vi "Initialize UDP Configuration.vi"(8 "error in (no error)":errorcluster, 11 "UDP Configuration in":refnum<class "UDP Configuration.lvclass">) -> (0 "error out":errorcluster, 3 "UDP Configuration out":refnum<class "UDP Configuration.lvclass">)   [LabVIEW 2017, in "UDP Transceiver.lvlib" / "UDP Configuration.lvclass"]
uses:
  UDP Configuration.lvclass
  C:/DSF/Core/Data Sharing Framework Core.lvlibp/Engine/Internal/Configuration Classes/Configuration/Configuration.lvclass
  UDP Configuration.lvclass/UDP Configuration.ctl
  DSF/Core/Data Sharing Framework Core.lvlibp/Engine/Internal/Configuration Classes/Configuration/Configuration.lvclass
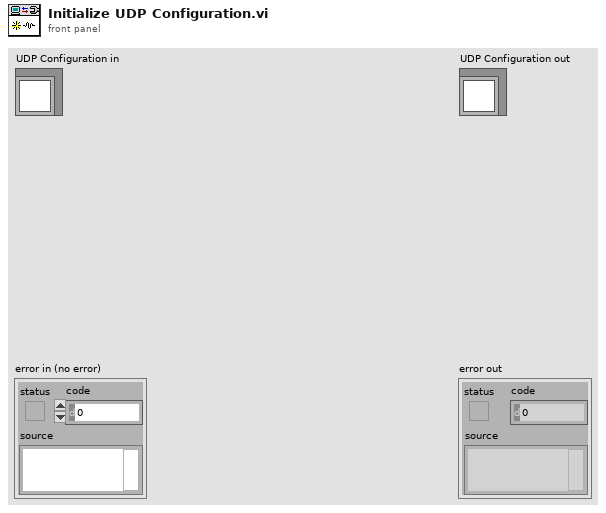
[diagram p1: front panel]
types:
  T1 = typedef "Data Sharing Framework Core.lvlibp/Data Sharing Framework Configuration.lvlib/DSF Settings Info.ctl" = cluster{"key":string, "value":string}[]
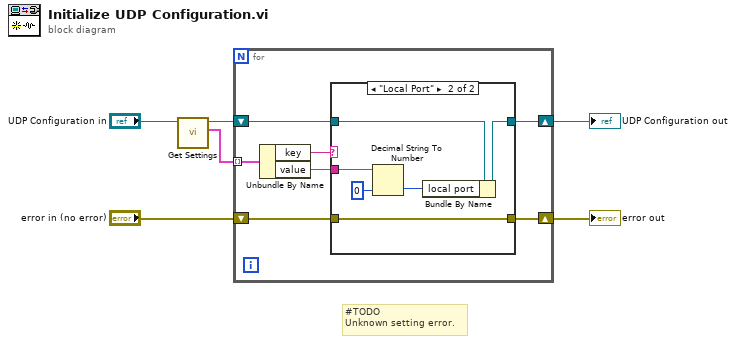
[diagram p0: block diagram]
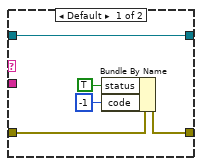
[diagram p2: hidden frame]
diagram:
  # "#TODO\nUnknown setting error."
  n1 = call "Get Settings.vi"("Configuration in"="UDP Configuration in") -> ("settings"=w5:T1, "Configuration out"=w4:refnum<class "UDP Configuration.lvclass">)  [unwired: 9 in]
  n2 = for {
    tunnel: w5 -> [w13] mode=indexing
    shift-right: [w9] -> w3
    shift-left: w4 -> [w10]
    shift-right: [w7] -> w1
    shift-left: "error in (no error)" -> [w8]
    n3 = Unbundle By Name(w13) -> ("key"=w12:string, "value"=w11:string)
    n4 = case shown="\"Local Port\"" w12 {
      tunnel: w11 -> [_ w23]
      tunnel: w10 -> [w18 w22]
      tunnel: [w18 w21] -> w9
      tunnel: w8 -> [w17 w19]
      tunnel: [w16 w19] -> w7
      frame Default {
        n5 = Bundle By Name(cluster=w17, "status"=TRUE, "code"=-1) -> (w16:errorcluster)
      }
      frame "Local Port" {
        n6 = Decimal String To Number(string=w23, default (0L)=u16 0 ("default (0 I32)")) -> (number=w20:u16)  [unwired: 1 in, 1 out]
        n7 = Bundle By Name(cluster=w22, "local port"=w20) -> (w21:refnum<class "UDP Configuration.lvclass">)
      }
    }
  }
  "error out" <- w1
  "UDP Configuration out" <- w3
